vi "Start VI.vi"(2 "error in":errorcluster, 3 "VI refnum":refnum<vi>[](array[refnum])) -> (0 "error out":errorcluster)   [LabVIEW 2011]
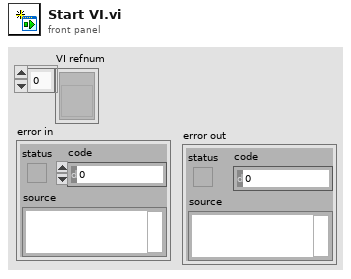
[diagram p1: front panel]
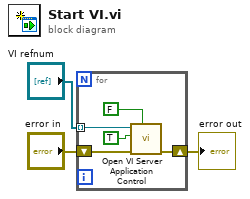
[diagram p0: block diagram]
diagram:
  n1 = for {
    tunnel: "VI refnum" -> [w8] mode=indexing
    shift-right: [w5] -> w1
    shift-left: "error in" -> [w4]
    n2 = call "Open VI Server Application Control.vi"("open front panel (F)"=FALSE ("Open Front Panel"), "error in (no error)"=w4, "run VI (F)"=TRUE ("Run VI"), "VI refnum"=w8) -> ("error out"=w5:errorcluster)  [unwired: 7 in]
  }
  "error out" <- w1
